vi "readVideoConfig.vi"(8 "error in (no error)":errorcluster) -> (0 "error out":errorcluster, 2 "Aiming Beam Config":T1, 3 "ini file path":path)   [LabVIEW 2020]
uses:
  AimingBeamVideoConfig.ctl
  <vilib>/Utility/config.llb/Read Key (I32).vi
  <vilib>/Utility/config.llb/Read Key (Boolean).vi
  <vilib>/Utility/config.llb/Read Key (Double).vi
  <vilib>/Utility/config.llb/NI_LVConfig.lvlib
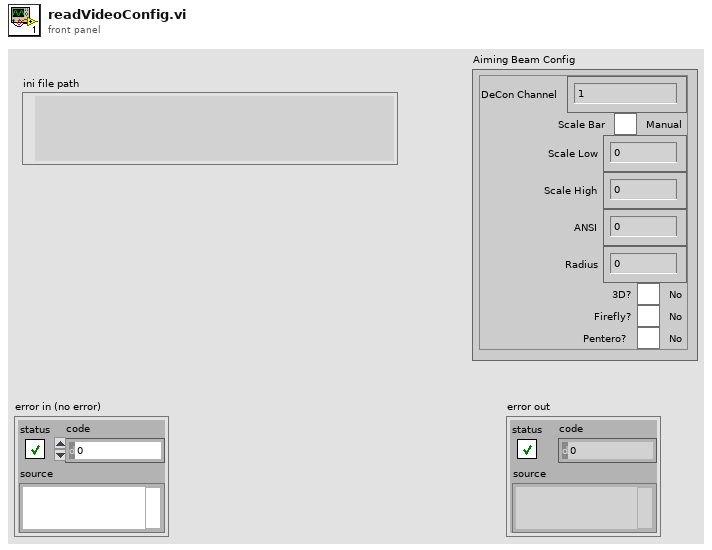
[diagram p1: front panel]
types:
  T1 = typedef "AimingBeamVideoConfig.ctl" = cluster{"DeCon Channel":enum16{"1", "2", "3"}, "Scale Bar":bool, "Scale Low":dbl, "Scale High":dbl, "ANSI":dbl, "Radius":dbl, "3D?":bool, "Firefly?":bool, "Pentero?":bool}
  T2 = typedef "NI_LVConfig.lvlib/Config Data RefNum.ctl" = refnum<k1>
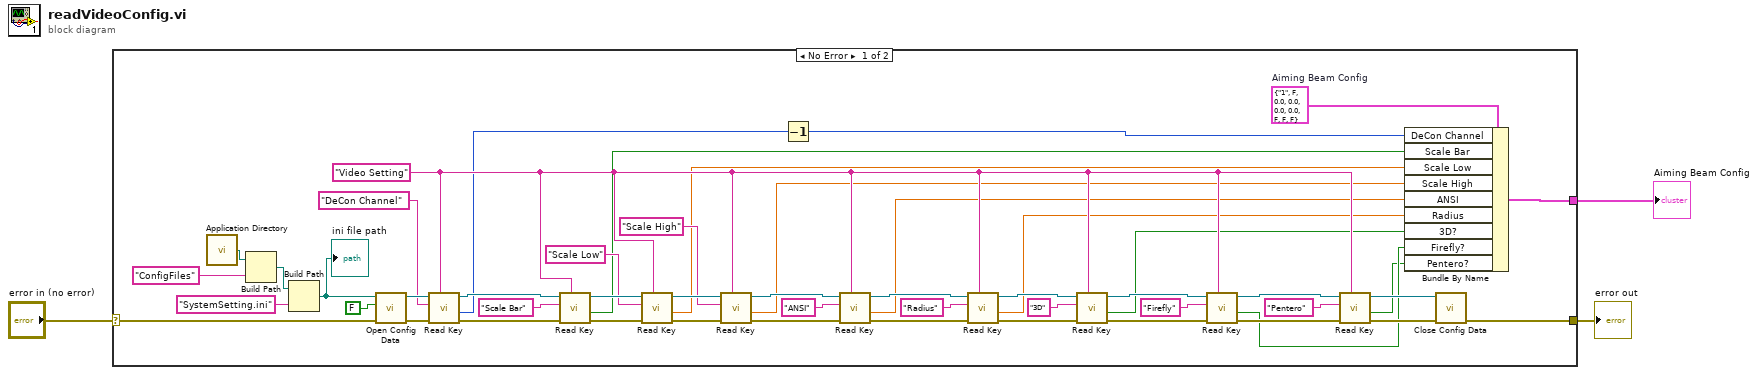
[diagram p0: block diagram]
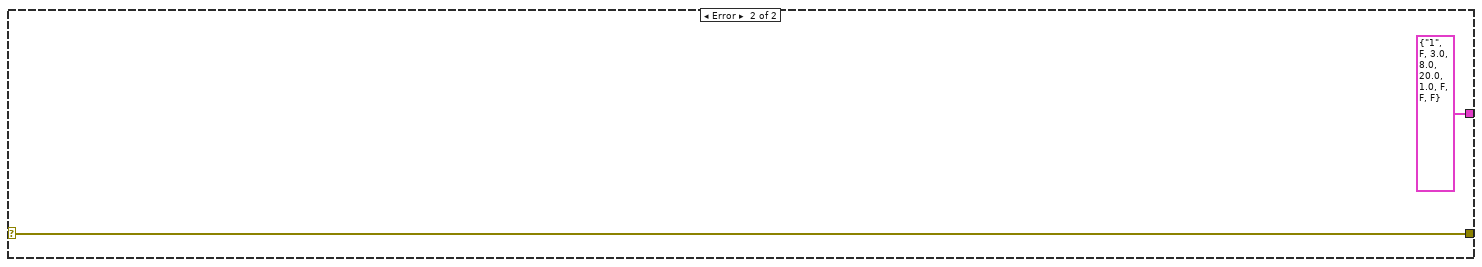
[diagram p2: hidden frame]
diagram:
  n1 = case shown="No Error" "error in (no error)" {
    selector: "error in (no error)" -> [w4 w54]
    tunnel: [w18 w54] -> w3
    tunnel: [w5 T1 {"DeCon Channel"=enum."1", "Scale Bar"=FALSE, "Scale Low"=3.0, "Scale High"=8.0, "ANSI"=20.0, "Radius"=1.0, "3D?"=FALSE, "Firefly?"=FALSE, "Pentero?"=FALSE} ("Aiming Beam Config")] -> w2
    frame No Error {
      w16 = T1 {"DeCon Channel"=enum."1", "Scale Bar"=FALSE, "Scale Low"=0.0, "Scale High"=0.0, "ANSI"=0.0, "Radius"=0.0, "3D?"=FALSE, "Firefly?"=FALSE, "Pentero?"=FALSE}  # Aiming Beam Config
      w17 = "Video Setting" ("section")
      n2 = call <vilib>:"Application Directory.vi"() -> ("Application Directory"=w52:path)
      n3 = Build Path(base path=w52, name or relative path="ConfigFiles") -> (appended path=w50:path)
      n4 = Build Path(base path=w50, name or relative path="SystemSetting.ini") -> (appended path=w48:path)
      "ini file path" <- w48
      n5 = call <vilib>:"Open Config Data.vi"("error in (no error)"=w4, "create file if necessary (T)"=FALSE, "configuration file path"=w48) -> ("error out"=w45:errorcluster, "refnum"=w47:T2)  [unwired: 6 in, 1 out]
      n6 = call-poly <vilib>:"Read Key.vi"("section"=w17, "error in (no error)"=w45, "key"="DeCon Channel", "refnum"=w47) -> ("error out"=w43:errorcluster, "value"=w14:i32, "refnum out"=w44:T2)  [unwired: 4 in, 1 out]
      n7 = call-poly <vilib>:"Read Key.vi"("section"=w17, "error in (no error)"=w43, "key"="Scale Bar", "refnum"=w44) -> ("error out"=w40:errorcluster, "value"=w13:bool, "refnum out"=w41:T2)  [unwired: 4 in, 1 out]
      n8 = call-poly <vilib>:"Read Key.vi"("section"=w17, "error in (no error)"=w40, "key"="Scale Low", "refnum"=w41) -> ("error out"=w36:errorcluster, "value"=w12:dbl, "refnum out"=w38:T2)  [unwired: 4 in, 1 out]
      n9 = call-poly <vilib>:"Read Key.vi"("section"=w17, "error in (no error)"=w36, "key"="Scale High", "refnum"=w38) -> ("error out"=w34:errorcluster, "value"=w11:dbl, "refnum out"=w35:T2)  [unwired: 4 in, 1 out]
      n10 = Decrement(x=w14) -> (x-1=w15:i32)
      n11 = call-poly <vilib>:"Read Key.vi"("section"=w17, "error in (no error)"=w34, "key"="ANSI", "refnum"=w35) -> ("error out"=w31:errorcluster, "value"=w10:dbl, "refnum out"=w32:T2)  [unwired: 4 in, 1 out]
      n12 = call-poly <vilib>:"Read Key.vi"("section"=w17, "error in (no error)"=w31, "key"="Radius", "refnum"=w32) -> ("error out"=w28:errorcluster, "value"=w9:dbl, "refnum out"=w29:T2)  [unwired: 4 in, 1 out]
      n13 = call-poly <vilib>:"Read Key.vi"("section"=w17, "error in (no error)"=w28, "key"="3D", "refnum"=w29) -> ("error out"=w25:errorcluster, "value"=w8:bool, "refnum out"=w26:T2)  [unwired: 4 in, 1 out]
      n14 = call-poly <vilib>:"Read Key.vi"("section"=w17, "error in (no error)"=w25, "key"="Firefly", "refnum"=w26) -> ("error out"=w22:errorcluster, "value"=w7:bool, "refnum out"=w23:T2)  [unwired: 4 in, 1 out]
      n15 = call-poly <vilib>:"Read Key.vi"("section"=w17, "error in (no error)"=w22, "key"="Pentero", "refnum"=w23) -> ("error out"=w19:errorcluster, "value"=w6:bool, "refnum out"=w20:T2)  [unwired: 4 in, 1 out]
      n16 = Bundle By Name(cluster=w16, "DeCon Channel"=w15, "Scale Bar"=w13, "Scale Low"=w12, "Scale High"=w11, "ANSI"=w10, "Radius"=w9, "3D?"=w8, "Firefly?"=w7, "Pentero?"=w6) -> (w5:T1)
      n17 = call <vilib>:"Close Config Data.vi"("error in (no error)"=w19, "refnum"=w20) -> ("error out"=w18:errorcluster)  [unwired: 8 in, 1 out]
    }
    frame Error {
    }
  }
  "error out" <- w3
  "Aiming Beam Config" <- w2
